vi "DSF.Engine.Plugin.Get Transceiver.vi"(11 "Plugin in":refnum<class "DSF.Engine.Plugin.lvclass">) -> (2 "Transceiver":refnum<class "DSF.Engine.Transceiver.lvclass">, 3 "Plugin out":refnum<class "DSF.Engine.Plugin.lvclass">)   [LabVIEW 2017, in "DSF.Engine.lvlib" / "DSF.Engine.Plugin.lvclass"]
uses:
  DSF.Engine.Plugin.lvclass
  Transceiver/DSF.Engine.Transceiver.lvclass
  DSF.Engine.Plugin.lvclass/DSF.Engine.Plugin.ctl
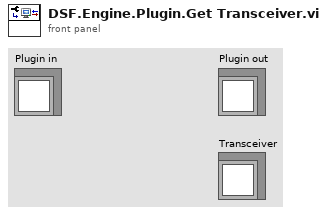
[diagram p1: front panel]
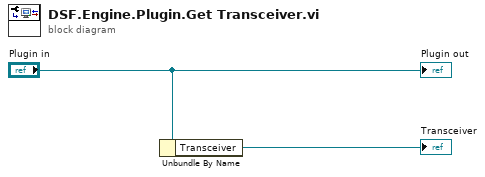
[diagram p0: block diagram]
diagram:
  n1 = Unbundle By Name("Plugin in") -> ("Transceiver"=→"Transceiver":refnum<class "DSF.Engine.Transceiver.lvclass">)
  "Plugin out" <- "Plugin in"
